vi "read_Object.vi"(0 "Interface_object in":refnum<class "DoorInterface.lvclass">, 3 "destroy Interface (T)":bool=TRUE, 5 "error in (no error)":errorcluster) -> (14 "Interface_object out":refnum<class "DoorInterface.lvclass">, 16 "Object":refnum<class>, 19 "error out":errorcluster)   [LabVIEW 2018, in "DoorInterface.lvclass"]
doc: "<b>Auto-created method</b>\n\nReturns object that can be downcast to specific class. The downcast must be done explicitly using node <b>To More Specific Class</b> and corresponding class constant. \n\nOptionally destroys instance of the Interface (but not instance of the class)."
uses:
  DoorInterface.lvclass
panel:
  # "Do not edit this method"
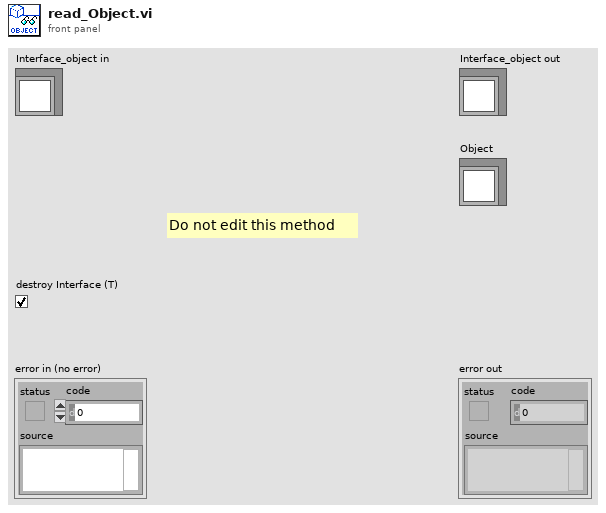
[diagram p1: front panel]
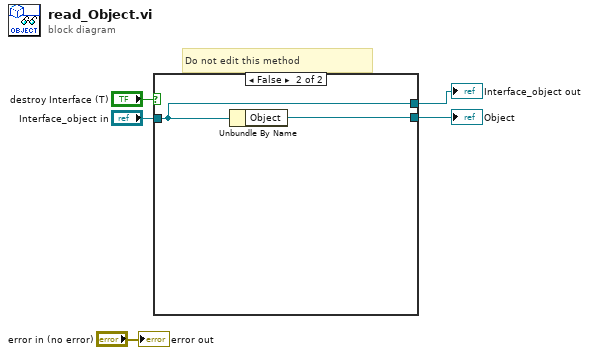
[diagram p0: block diagram]
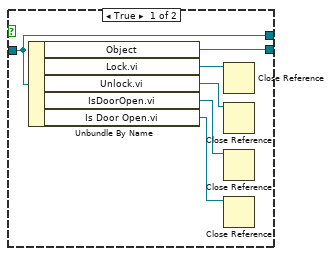
[diagram p2: hidden frame]
diagram:
  # "Do not edit this method"
  n1 = case shown="False" "destroy Interface (T)" {
    tunnel: [w11 w13] -> w3
    tunnel: "Interface_object in" -> [w11 w13]
    tunnel: [w10 w12] -> w1
    frame True {
      n2 = Unbundle By Name(w11) -> ("Object"=w10:refnum<class>, "Lock.vi"=w9:refnum<vi>, "Unlock.vi"=w8:refnum<vi>, "IsDoorOpen.vi"=w7:refnum<vi>, "Is Door Open.vi"=w6:refnum<vi>)
      n3 = Close Reference(reference=w9) -> ()  [unwired: 1 in, 1 out]
      n4 = Close Reference(reference=w8) -> ()  [unwired: 1 in, 1 out]
      n5 = Close Reference(reference=w7) -> ()  [unwired: 1 in, 1 out]
      n6 = Close Reference(reference=w6) -> ()  [unwired: 1 in, 1 out]
    }
    frame False {
      n7 = Unbundle By Name(w13) -> ("Object"=w12:refnum<class>)
    }
  }
  "Interface_object out" <- w3
  "Object" <- w1
  "error out" <- "error in (no error)"
